vi "Write Frame Crop Utility.vi"(6 "list only?":bool, 8 "error in (no error)":errorcluster, 9 "export to TIFFs?":bool, 10 "Starting frame number":u32, 11 "Frame Grabber Data In in":T1={"Camera Session"="", "Frame"=refnum, "AVI Refnum"=refnum, "Codecs"=[], "Frame number"=0, "Tracking File Refnum"=refnum, "Tick Count"=0, "Probe Object"=refnum, "Playback Probe Data"=[], "Rigid Body"={"Position"={"x (mm)"=0.0, "y (mm)"=0.0, "z (mm)"=0.0}, "Orientation"={"Pitch (rad)"=0.0, "Yaw (rad)"=0.0, "Roll (rad)"=0.0}, "Quaternion"={"qx"=0.0, "qy"=0.0, "qz"=0.0, "qw"=0.0}, "Tracked?"=FALSE}, "Total no frames playback"=0, "Video FPS"=0.0, "Camera connected?"=FALSE, "Scene"=refnum, "Cropped Frame"=refnum, "Tracker FPS"=0.0, "Crop ROI"=[], "Presentation Values"=[], "Elapsed time (ms)"=0, "Camera frames playback"=0, "Refnums"={"Live Refnum"=refnum, "Record Refnum"=refnum, "Playback Refnum"=refnum, "Frame Slider Refnum"=refnum, "Pause Refnum"=refnum, "Home Refnum"=refnum, "Set Crop Refnum"=refnum, "Clear Crop Refnum"=refnum, "stop refnum"=refnum, "Playback Rate Refnum"=refnum, "Presentation Refnum"=refnum, "Crop Time Frame Slider Refnum"=refnum, "Cancel Save Refnum"=refnum, "Reverse Playback Refnum"=refnum, "Recording Settings Refnum"=refnum, "Continuous Playback Refnum"=refnum, "Annotation Refnum"=refnum, "Export All Refnum"=refnum, "Export List Refnum"=refnum, "Fill List Refnum"=refnum, "Save Crop Refnum"=refnum, "Skip Forward Refnum"=refnum, "Skip Backward Refnum"=refnum, "Single Annotation Refnum"=refnum, "Load Video Refnum"=refnum, "Set Start Refnum"=refnum, "Set End Refnum"=refnum, "Add to List Refnum"=refnum, "List of Annotations Refnum"=refnum, "Camera Frame Refnum"=refnum, "Load Image Refnum"=refnum, "Saving Refnum"=refnum}, "Dimensions"={"Probe Dimensions"={"Probe Width"=0.0, "Probe Depth"=1.0, "Probe Height"=0.0}, "Room Dimensions"={"Room Width"=0.0, "Room Depth"=0.0, "Room Height"=0.0}}, "Playback Data As Strings"=[], "Cropped Tracking File Refnum"=refnum, "Cropped AVI Refnum"=refnum, "Header"=[], "Total euclidian distance"=0.0, "Annotation File Path"=path "", "Playback File Path"=path "", "Size per frame"=0.0, "Ground Truth File Refnum"=refnum, "Annotation Array"=[], "Annotation TIFFs Folder"=path "", "overwriting open file?"=FALSE, "Image Sequence"=[], "Video/Image Flag"=enum."Playback Video Frame", "Image sequence?"=FALSE, "Image sequence filenames"=[]}) -> (0 "error out":errorcluster, 1 "annotated camera frame number":i32, 2 "Cancel save?":bool, 3 "Frame Grabber Data out":T1={"Camera Session"="", "Frame"=refnum, "AVI Refnum"=refnum, "Codecs"=[], "Frame number"=0, "Tracking File Refnum"=refnum, "Tick Count"=0, "Probe Object"=refnum, "Playback Probe Data"=[], "Rigid Body"={"Position"={"x (mm)"=0.0, "y (mm)"=0.0, "z (mm)"=0.0}, "Orientation"={"Pitch (rad)"=0.0, "Yaw (rad)"=0.0, "Roll (rad)"=0.0}, "Quaternion"={"qx"=0.0, "qy"=0.0, "qz"=0.0, "qw"=0.0}, "Tracked?"=FALSE}, "Total no frames playback"=0, "Video FPS"=0.0, "Camera connected?"=FALSE, "Scene"=refnum, "Cropped Frame"=refnum, "Tracker FPS"=0.0, "Crop ROI"=[], "Presentation Values"=[], "Elapsed time (ms)"=0, "Camera frames playback"=0, "Refnums"={"Live Refnum"=refnum, "Record Refnum"=refnum, "Playback Refnum"=refnum, "Frame Slider Refnum"=refnum, "Pause Refnum"=refnum, "Home Refnum"=refnum, "Set Crop Refnum"=refnum, "Clear Crop Refnum"=refnum, "stop refnum"=refnum, "Playback Rate Refnum"=refnum, "Presentation Refnum"=refnum, "Crop Time Frame Slider Refnum"=refnum, "Cancel Save Refnum"=refnum, "Reverse Playback Refnum"=refnum, "Recording Settings Refnum"=refnum, "Continuous Playback Refnum"=refnum, "Annotation Refnum"=refnum, "Export All Refnum"=refnum, "Export List Refnum"=refnum, "Fill List Refnum"=refnum, "Save Crop Refnum"=refnum, "Skip Forward Refnum"=refnum, "Skip Backward Refnum"=refnum, "Single Annotation Refnum"=refnum, "Load Video Refnum"=refnum, "Set Start Refnum"=refnum, "Set End Refnum"=refnum, "Add to List Refnum"=refnum, "List of Annotations Refnum"=refnum, "Camera Frame Refnum"=refnum, "Load Image Refnum"=refnum, "Saving Refnum"=refnum}, "Dimensions"={"Probe Dimensions"={"Probe Width"=0.0, "Probe Depth"=1.0, "Probe Height"=0.0}, "Room Dimensions"={"Room Width"=0.0, "Room Depth"=0.0, "Room Height"=0.0}}, "Playback Data As Strings"=[], "Cropped Tracking File Refnum"=refnum, "Cropped AVI Refnum"=refnum, "Header"=[], "Total euclidian distance"=0.0, "Annotation File Path"=path "", "Playback File Path"=path "", "Size per frame"=0.0, "Ground Truth File Refnum"=refnum, "Annotation Array"=[], "Annotation TIFFs Folder"=path "", "overwriting open file?"=FALSE, "Image Sequence"=[], "Video/Image Flag"=enum."Playback Video Frame", "Image sequence?"=FALSE, "Image sequence filenames"=[]})   [LabVIEW 2017]
uses:
  Controls/Frame Grabber Data.ctl
  <vilib>/userdefined/High Color/IMAQdx.ctl
  <vilib>/vision/Image Controls.llb/IMAQ Image.ctl
  <vilib>/vision/Avi.llb/IMAQ AVI2 Refnum.ctl
  Controls/Rigid Body Info.ctl
  Controls/Position.ctl
  Controls/Orientation.ctl
  Controls/Refnums.ctl
  Controls/Recording Settings.ctl
  Controls/Operator Settings.ctl
  Controls/Operator.ctl
  Controls/Patient Settings.ctl
  Controls/Dimensions.ctl
  Controls/Room Dimensions.ctl
  Controls/Crop Video State.ctl
  <vilib>/vision/NI_Vision_Development_Module.lvlib
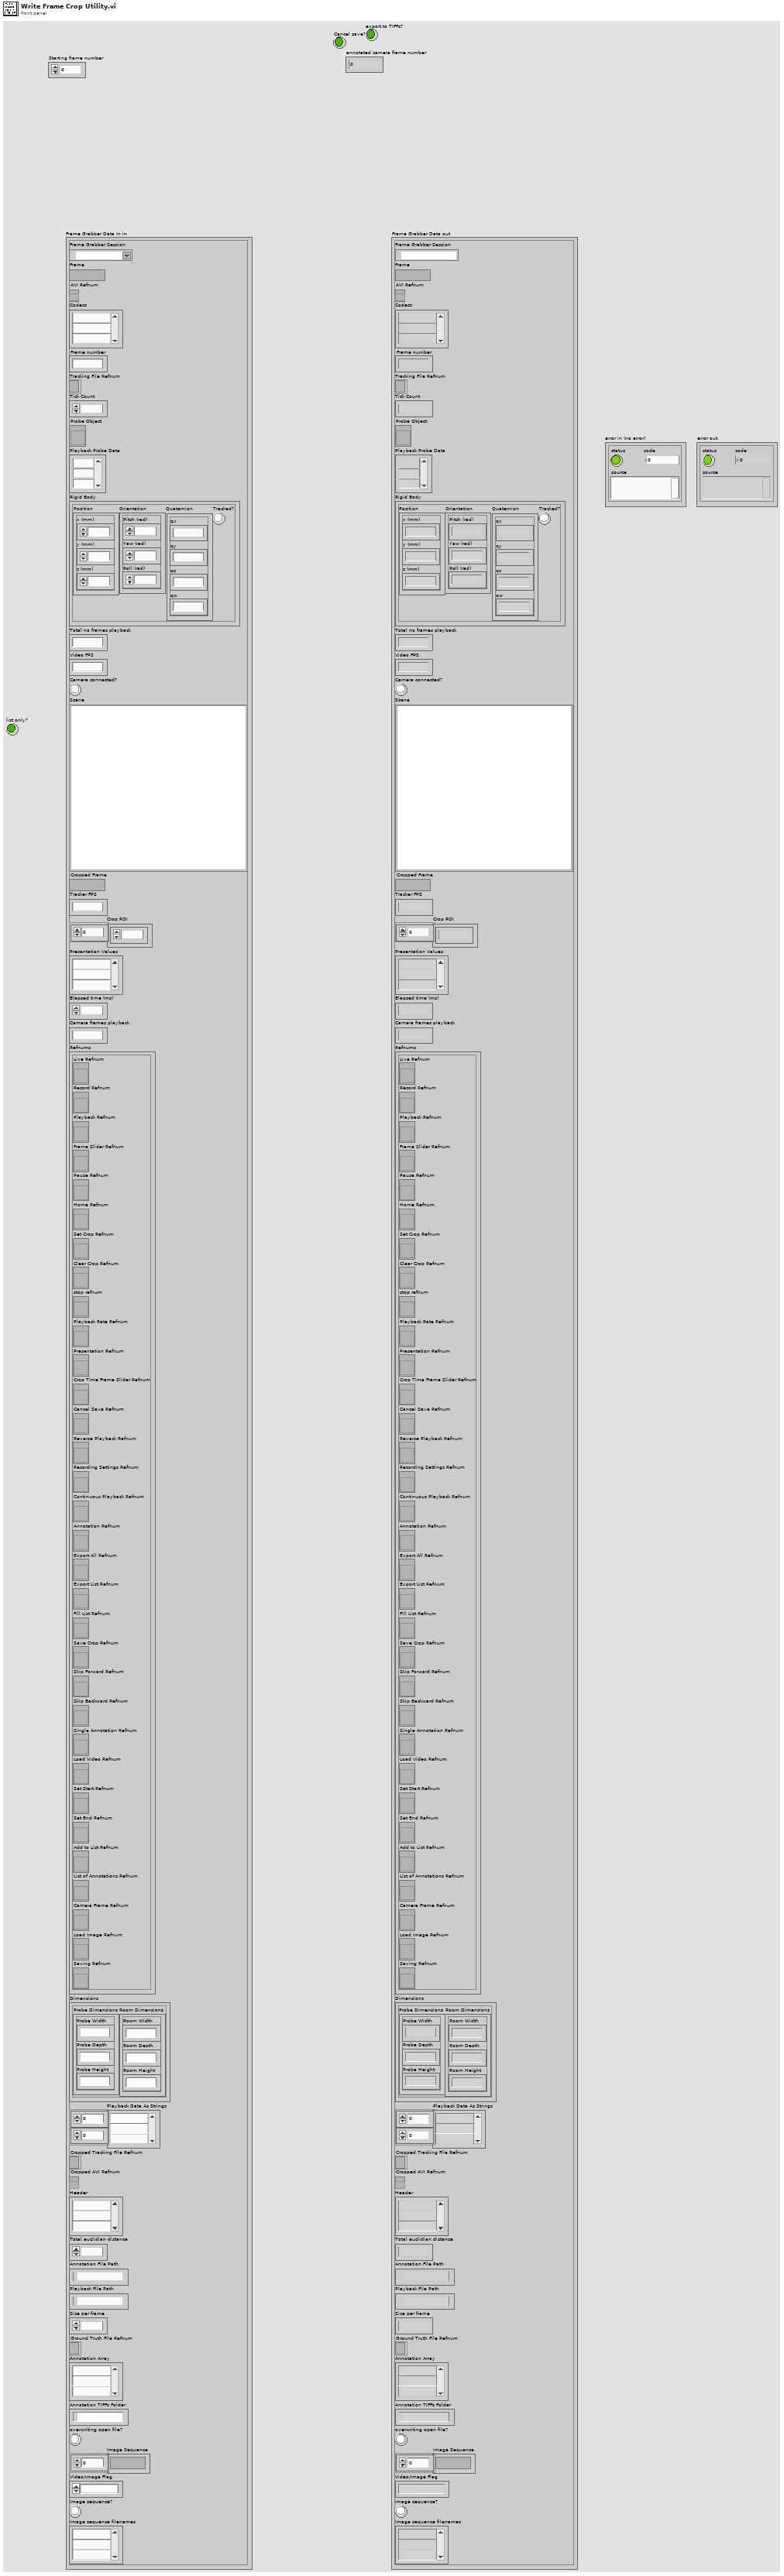
[diagram p1: front panel]
types:
  T1 = typedef "Frame Grabber Data.ctl" = cluster{"Camera Session":T2, "Frame":T3, "AVI Refnum":T4, "Codecs":string[], "Frame number":u32, "Tracking File Refnum":refnum<file>, "Tick Count":u32, "Probe Object":refnum<vi>, "Playback Probe Data":dbl[][], "Rigid Body":T5, "Total no frames playback":i32, "Video FPS":dbl, "Camera connected?":bool, "Scene":refnum<vi>, "Cropped Frame":T3, "Tracker FPS":dbl, "Crop ROI":i32[], "Presentation Values":string[], "Elapsed time (ms)":u32, "Camera frames playback":u32, "Refnums":T8, "Dimensions":T9, "Playback Data As Strings":string[][], "Cropped Tracking File Refnum":refnum<file>, "Cropped AVI Refnum":T4, "Header":string[], "Total euclidian distance":dbl, "Annotation File Path":path, "Playback File Path":path, "Size per frame":dbl, "Ground Truth File Refnum":refnum<file>, "Annotation Array":string[], "Annotation TIFFs Folder":path, "overwriting open file?":bool, "Image Sequence":T3[], "Video/Image Flag":T11, "Image sequence?":bool, "Image sequence filenames":string[]}
  T2 = typedef "IMAQdx.ctl" = refnum<k21>
  T3 = typedef "IMAQ Image.ctl" = refnum<image>
  T4 = typedef "IMAQ AVI2 Refnum.ctl" = refnum<k20>
  T5 = typedef "Rigid Body Info.ctl" = cluster{"Position":T6, "Orientation":T7, "Quaternion":cluster{"qx":sgl, "qy":sgl, "qz":sgl, "qw":sgl}, "Tracked?":bool}
  T6 = typedef "Position.ctl" = cluster{"x (mm)":sgl, "y (mm)":sgl, "z (mm)":sgl}
  T7 = typedef "Orientation.ctl" = cluster{"Pitch (rad)":sgl, "Yaw (rad)":sgl, "Roll (rad)":sgl}
  T8 = typedef "Refnums.ctl" = cluster{"Live Refnum":refnum<vi>, "Record Refnum":refnum<vi>, "Playback Refnum":refnum<vi>, "Frame Slider Refnum":refnum<vi>, "Pause Refnum":refnum<vi>, "Home Refnum":refnum<vi>, "Set Crop Refnum":refnum<vi>, "Clear Crop Refnum":refnum<vi>, "stop refnum":refnum<vi>, "Playback Rate Refnum":refnum<vi>, "Presentation Refnum":refnum<vi>, "Crop Time Frame Slider Refnum":refnum<vi>, "Cancel Save Refnum":refnum<vi>, "Reverse Playback Refnum":refnum<vi>, "Recording Settings Refnum":refnum<vi>, "Continuous Playback Refnum":refnum<vi>, "Annotation Refnum":refnum<vi>, "Export All Refnum":refnum<vi>, "Export List Refnum":refnum<vi>, "Fill List Refnum":refnum<vi>, "Save Crop Refnum":refnum<vi>, "Skip Forward Refnum":refnum<vi>, "Skip Backward Refnum":refnum<vi>, "Single Annotation Refnum":refnum<vi>, "Load Video Refnum":refnum<vi>, "Set Start Refnum":refnum<vi>, "Set End Refnum":refnum<vi>, "Add to List Refnum":refnum<vi>, "List of Annotations Refnum":refnum<vi>, "Camera Frame Refnum":refnum<vi>, "Load Image Refnum":refnum<vi>, "Saving Refnum":refnum<vi>}
  T9 = typedef "Dimensions.ctl" = cluster{"Probe Dimensions":cluster{"Probe Width":sgl, "Probe Depth":sgl, "Probe Height":sgl}, "Room Dimensions":T10}
  T10 = typedef "Room Dimensions.ctl" = cluster{"Room Width":dbl, "Room Depth":dbl, "Room Height":dbl}
  T11 = typedef "Crop Video State.ctl" = enum16{"Init", "Wait", "Load Image", "Load Video", "Play/Pause", "Playback Video Frame", "Display Image", "Save Image Sequence", "Save Video", "Export List", "Export All", "Close", "Set Crop Area", "Reset Crop Area", "Crop Inside", "Crop Outside", "Multi-Crop", "Re-Open Files", "Annotate Frame", "Annotate Clip", "Add to List", "Fill List", "Set Start", "Set End", "Error Handling", "Shutdown"}
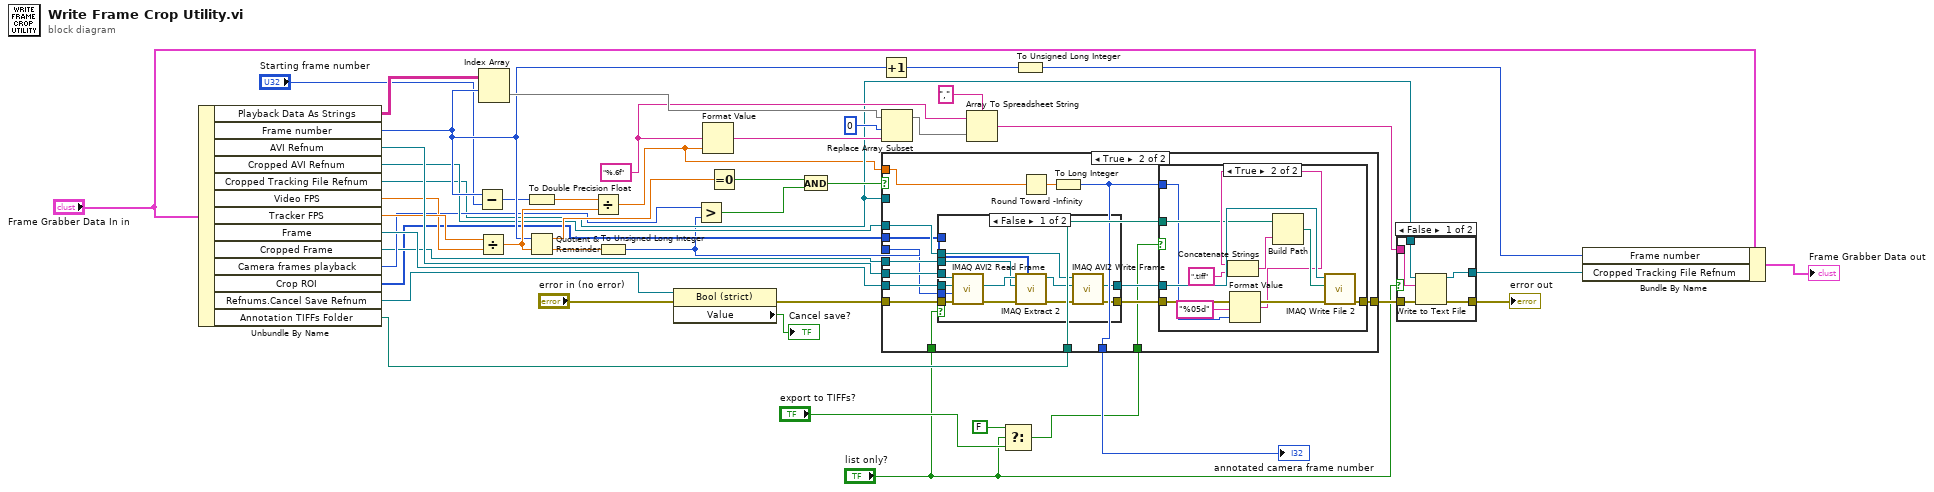
[diagram p0: block diagram]
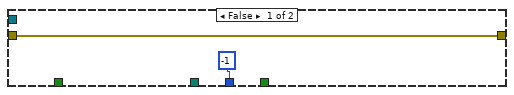
[diagram p3: hidden frame]
diagram:
  w23 = "%.6f" ("format string")
  n1 = Unbundle By Name("Frame Grabber Data In in") -> ("Playback Data As Strings"=w34:string[][], "Frame number"=w29:u32, "AVI Refnum"=w37:T4, "Cropped AVI Refnum"=w24:T4, "Cropped Tracking File Refnum"=w13:refnum<file>, "Video FPS"=w35:dbl, "Tracker FPS"=w36:dbl, "Frame"=w38:T3, "Cropped Frame"=w19:T3, "Camera frames playback"=w21:u32, "Crop ROI"=w18:i32[], "Refnums.Cancel Save Refnum"=w16:refnum<vi>, "Annotation TIFFs Folder"=w7:path)
  n2 = Subtract(x=w29, y="Starting frame number") -> (x-y=w11:u32)
  n3 = Divide(x=w36, y=w35) -> (x/y=w42:dbl)
  n4 = Index Array(array=w34, index (row)=w29) -> (element=w33:string[])  [unwired: 1 in]
  n5 = To Double Precision Float(number=w11) -> (double precision float=w41:dbl)
  n6 = Quotient & Remainder(x=w29, y=w42) -> (x-y*floor(x/y)=w43:dbl, floor(x/y)=w39:dbl)
  n7 = Divide(x=w41, y=w42) -> (x/y=w5:dbl)
  n8 = To Unsigned Long Integer(number=w39) -> (unsigned 32bit integer=w12:u32)
  n9 = property class="Bool (strict)"(reference=w16, error in="error in (no error)") -> (error out=w15:errorcluster, "Value"=→"Cancel save?":bool)  [unwired: 1 out]
  n10 = Greater?(x=w21, y=w12) -> (0:w20:bool)
  n11 = Format Value(format string=w23, value (0)=w5) -> (output string=w31:string)  [unwired: 1 in]
  n12 = Equal To 0?(x=w43) -> (x = 0?=w40:bool)
  n13 = And(x=w40, y=w20) -> (x .and. y?=w22:bool)
  n14 = Increment(x=w29) -> (x+1=w44:u32)
  n15 = Replace Array Subset(array=w33, new element=w31, index=0) -> (w27:string[])
  n16 = Array To Spreadsheet String(delimiter (Tab)=",", array=w27, 3:w23) -> (spreadsheet string=w25:string)
  n17 = Select(t=FALSE, s="list only?", f="export to TIFFs?") -> (s? t:f=w2:bool)
  n18 = case shown="True" w22 {
    tunnel: [w48 w57] -> w46
    tunnel: w15 -> [w48 w64]
    tunnel: w38 -> [_ w63]
    tunnel: w37 -> [_ w62]
    tunnel: w12 -> [_ w54]
    tunnel: w24 -> [_ w61]
    tunnel: w19 -> [_ w60]
    tunnel: w18 -> [_ w59]
    tunnel: w13 -> [_ _]
    tunnel: w2 -> [_ w55]
    tunnel: [-1 w50] -> w10
    tunnel: w7 -> [_ w53]
    tunnel: w5 -> [_ w52]
    tunnel: "list only?" -> [_ w49]
    frame False {
    }
    frame True {
      n19 = case shown="False" w49 {
        tunnel: w64 -> [w77 w78]
        tunnel: w63 -> [w76 w79]
        tunnel: w62 -> [w75 _]
        tunnel: w61 -> [w74 _]
        tunnel: w60 -> [w70 _]
        tunnel: w59 -> [w69 _]
        tunnel: [w68 w78] -> w58
        tunnel: [w66 w79] -> w56
        tunnel: w54 -> [w65 _]
        frame False {
          n20 = call "IMAQ AVI2 Read Frame"("error in (no error)"=w77, "Frame Number"=w65, "Image"=w76, "AVI Refnum"=w75) -> ("error out"=w73:errorcluster, "Image Out"=w71:T3)  [unwired: 5 in, 1 out]
          n21 = call "IMAQ Extract 2"("Optional Rectangle"=w69, "error in (no error)"=w73, "Image Dst"=w70, "Image Src"=w71) -> ("error out"=w72:errorcluster, "Image Dst Out"=w67:T3)  [unwired: 6 in]
          n22 = call "IMAQ AVI2 Write Frame"("error in (no error)"=w72, "Image"=w67, "AVI Refnum"=w74) -> ("error out"=w68:errorcluster, "Image Out (duplicate)"=w66:T3)  [unwired: 6 in, 1 out]
        }
        frame True {
        }
      }
      n23 = Round Toward -Infinity(1:w52) -> (0:w51:dbl)
      n24 = To Long Integer(number=w51) -> (32bit integer=w50:i32)
      n25 = case shown="True" w55 {
        tunnel: w58 -> [w80 w90]
        tunnel: [w80 w89] -> w57
        tunnel: w56 -> [_ w88]
        tunnel: w53 -> [_ w82]
        tunnel: w50 -> [_ w81]
        frame False {
        }
        frame True {
          n26 = Format Value(format string="%05d", value (0)=w81) -> (output string=w83:string)  [unwired: 1 in]
          n27 = Concatenate Strings(w83, ".tiff") -> (w86:string)
          n28 = Build Path(base path=w82, name or relative path=w86) -> (appended path=w85:path)
          n29 = call-poly "IMAQ Write File 2"("error in (no error)"=w90, "File Path"=w85, "Image"=w88) -> ("error out"=w89:errorcluster)  [unwired: 7 in, 1 out]
        }
      }
    }
  }
  "annotated camera frame number" <- w10
  n30 = To Unsigned Long Integer(number=w44) -> (unsigned 32bit integer=w30:u32)
  n31 = case shown="False" "list only?" {
    tunnel: w46 -> [w95 w97]
    tunnel: [w94 w96] -> w45
    tunnel: [w93 w97] -> w28
    tunnel: w25 -> [w92 _]
    tunnel: w13 -> [w91 w96]
    frame False {
      n32 = Write to Text File(file (use dialog)=w91, text=w92, error in=w95) -> (refnum out=w94:refnum<file>, error out=w93:errorcluster)  [unwired: 1 in, 1 out]
    }
    frame True {
    }
  }
  "error out" <- w28
  n33 = Bundle By Name(cluster="Frame Grabber Data In in", "Frame number"=w30, "Cropped Tracking File Refnum"=w45) -> (→"Frame Grabber Data out":T1)
